vi "Read SA Pin.vi"(8 "error in (no error)":errorcluster, 11 "WCDMA_OBW in":refnum<class "WCDMA_OBW.lvclass">=refnum) -> (0 "error out":errorcluster, 2 "SA Pin":string, 3 "WCDMA_OBW out":refnum<class "WCDMA_OBW.lvclass">)   [LabVIEW 2016, in "SeqAuto Evaluations.lvlib" / "WCDMA_OBW.lvclass"]
uses:
  WCDMA_OBW.lvclass
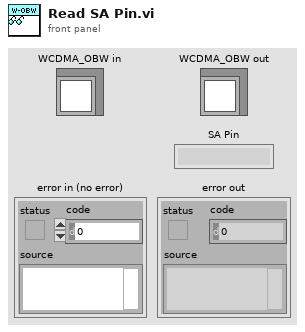
[diagram p1: front panel]
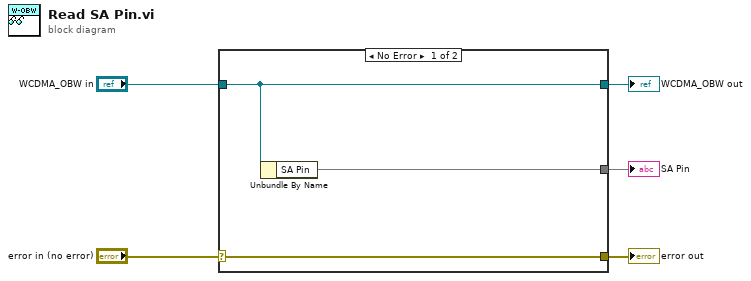
[diagram p0: block diagram]
diagram:
  n1 = case shown="No Error" "error in (no error)" {
    selector: "error in (no error)" -> [w8 w9]
    tunnel: [w8 w9] -> w4
    tunnel: [w7 w10] -> w2
    tunnel: "WCDMA_OBW in" -> [w7 w10]
    tunnel: [w6 _] -> w1
    frame No Error {
      n2 = Unbundle By Name(w7) -> ("SA Pin"=w6)
    }
    frame Error {
    }
  }
  "error out" <- w4
  "WCDMA_OBW out" <- w2
  "SA Pin" <- w1
